vi "t3_parse_stream.vi"(6 "first_batch?":bool, 7 "Last_sync":cluster{"sync_counter":i32, "sync_time":dbl}, 8 "Error In":errorcluster, 9 "stamps":dbl[](array[numeric]), 10 "channels":dbl[](array[numeric]), 11 "reference_channel":dbl) -> (0 "Error In 2":errorcluster, 1 "count_timestamps":dbl[](array[numeric]), 2 "n_sync array":dbl[](array[numeric]), 3 "channels":dbl[](array[numeric]), 4 "first_batch?":bool, 5 "last_sync_out":cluster{"sync_counter":i32, "sync_time":dbl})   [LabVIEW 2018]
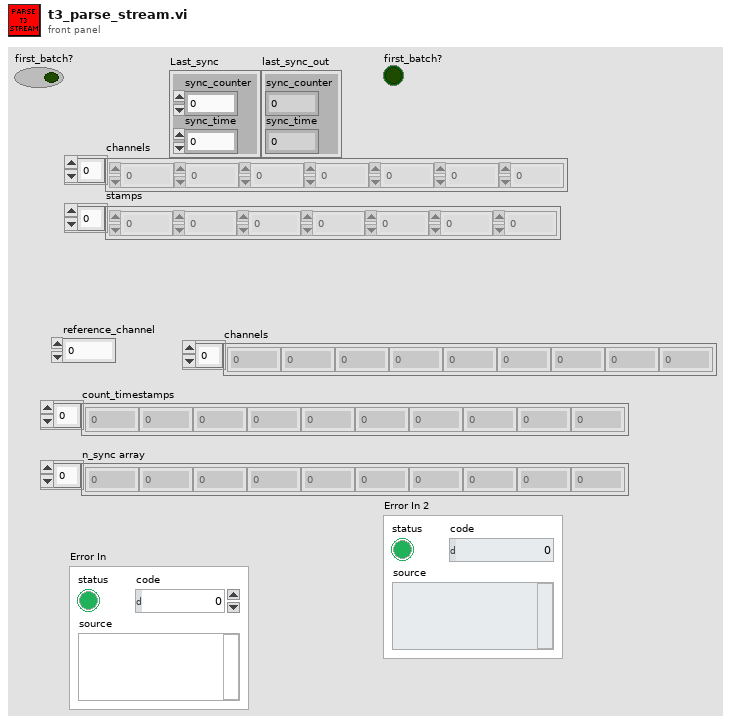
[diagram p1: front panel]
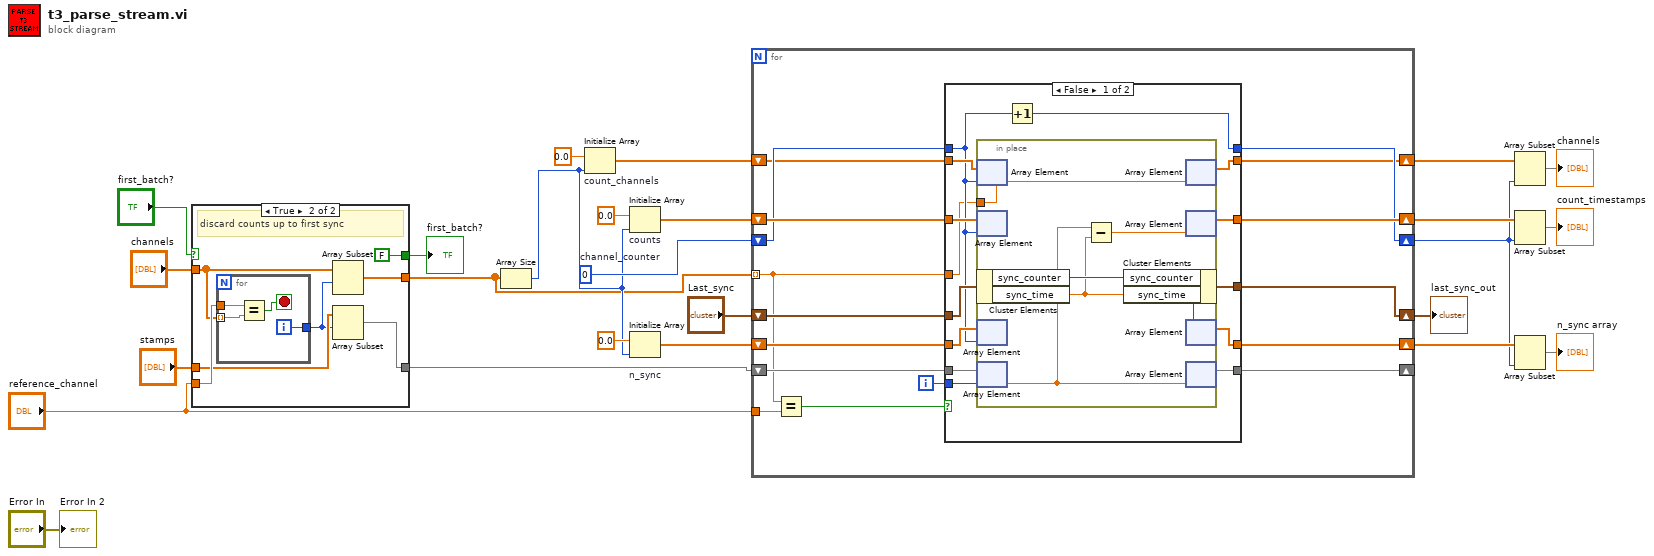
[diagram p0: block diagram]
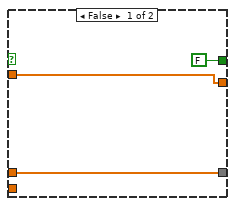
[diagram p2: hidden frame]
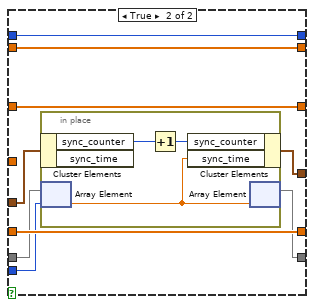
[diagram p3: hidden frame]
diagram:
  w21 = 0  # channel_counter
  n1 = case shown="True" "first_batch?" {
    tunnel: "reference_channel" -> [_ w35]
    tunnel: "channels" -> [w28 w34]
    tunnel: [w28 w33] -> w4
    tunnel: "stamps" -> [w27 w32]
    tunnel: [w27 w30] -> w2
    tunnel: [FALSE FALSE] -> w1
    frame False {
    }
    frame True {
      # "discard counts up to first sync"
      n2 = for {
        tunnel: w35 -> [w38]
        tunnel: w34 -> [w39] mode=indexing
        tunnel: [w37] -> w31
        i -> [w37]
        stop <- w36 stop-if-true
        n3 = Equal?(x=w38, y=w39) -> (x = y?=w36:bool)
      }
      n4 = Array Subset(array=w34, index=w31) -> (w33:dbl[])  [unwired: 1 in]
      n5 = Array Subset(array=w32, index=w31) -> (w30:dbl[])  [unwired: 1 in]
    }
  }
  "first_batch?" <- w1
  n6 = Array Size(array=w4) -> (size(s)=w15:i32)
  n7 = Initialize Array "count_channels"(0.0 ("element"), w15) -> (w14:dbl[])
  n8 = Initialize Array "counts"(0.0 ("element"), w15) -> (w22:dbl[])
  n9 = Initialize Array "n_sync"(0.0 ("element"), w15) -> (w24:dbl[])
  n10 = for {
    tunnel: w4 -> [w41] mode=indexing
    shift-right: [w46] -> _
    shift-left: w2 -> [w47]
    tunnel: "reference_channel" -> [w55]
    shift-right: [w52] -> w20
    shift-left: w22 -> [w54]
    shift-right: [w51] -> w19
    shift-left: w24 -> [w53]
    shift-right: [w49] -> w9
    shift-left: "Last_sync" -> [w50]
    shift-right: [w44] -> w12
    shift-left: w21 -> [w45]
    shift-right: [w40] -> w13
    shift-left: w14 -> [w42]
    i -> [w48]
    n11 = Equal?(x=w41, y=w55) -> (x = y?=w43:bool)
    n12 = case shown="False" w43 {
      tunnel: w54 -> [w66 w83]
      tunnel: w53 -> [w68 w82]
      tunnel: [w63 w83] -> w52
      tunnel: [w61 w82] -> w51
      tunnel: w50 -> [w69 w81]
      tunnel: [w67 w77] -> w49
      tunnel: w48 -> [w65 w80]
      tunnel: w47 -> [w64 w79]
      tunnel: [w62 w78] -> w46
      tunnel: w45 -> [w58 w76]
      tunnel: [w60 w76] -> w44
      tunnel: w42 -> [w59 w75]
      tunnel: w41 -> [w57 _]
      tunnel: [w56 w75] -> w40
      frame False {
        n13 = in-place {
          in-place-border: w57 -> [w73]
          n14 = in-place-array #1(w59, w58) -> ()  [unwired: 1 out]
          n15 = in-place-array #2(w66, w58) -> ()  [unwired: 1 out]
          n16 = in-place-cluster #3(w69) -> ("sync_counter"=w74:i32, "sync_time"=w70:dbl)
          n17 = in-place-array #4(w68, w58) -> ()  [unwired: 1 out]
          n18 = in-place-array #5(w64, w65) -> (w71:dbl)
          n19 = Subtract(x=w71, y=w70) -> (x-y=w72:dbl)
          n20 = in-place-cluster #3("sync_counter"=w74, "sync_time"=w70) -> (w67:cluster{"sync_counter":i32, "sync_time":dbl})
          n21 = in-place-array #1(w73) -> (w56:dbl[])  [unwired: 1 out]
          n22 = in-place-array #2(w72) -> (w63:dbl[])  [unwired: 1 out]
          n23 = in-place-array #4(w74) -> (w61:dbl[])  [unwired: 1 out]
          n24 = in-place-array #5(w71) -> (w62:dbl[])  [unwired: 1 out]
        }
        n25 = Increment(x=w58) -> (x+1=w60:i32)
      }
      frame True {
        n26 = in-place {
          n27 = in-place-cluster #6(w81) -> ("sync_counter"=w86:i32)  [unwired: 1 out]
          n28 = in-place-array #7(w79, w80) -> (w84:dbl)
          n29 = Increment(x=w86) -> (x+1=w85:i32)
          n30 = in-place-cluster #6("sync_counter"=w85, "sync_time"=w84) -> (w77:cluster{"sync_counter":i32, "sync_time":dbl})
          n31 = in-place-array #7(w84) -> (w78:dbl[])  [unwired: 1 out]
        }
      }
    }
  }
  "last_sync_out" <- w9
  n32 = Array Subset(array=w13, length=w12) -> (→"channels":dbl[])  [unwired: 1 in]
  n33 = Array Subset(array=w20, length=w12) -> (→"count_timestamps":dbl[])  [unwired: 1 in]
  n34 = Array Subset(array=w19, length=w12) -> (→"n_sync array":dbl[])  [unwired: 1 in]
  "Error In 2" <- "Error In"
